vi "Stopt VI Event.vi"(2 "error in":errorcluster, 3 "VI refnum":refnum<vi>[](array[refnum])) -> (0 "error out":errorcluster)   [LabVIEW 2012]
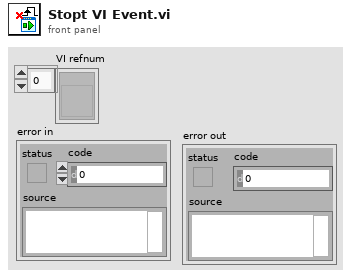
[diagram p1: front panel]
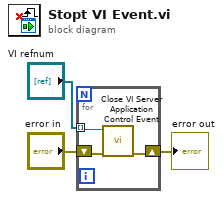
[diagram p0: block diagram]
diagram:
  n1 = for {
    tunnel: "VI refnum" -> [w6] mode=indexing
    shift-right: [w4] -> w1
    shift-left: "error in" -> [w5]
    n2 = call "Close VI Server Application Control Event.vi"("error in (no error)"=w5, "VI refnum"=w6) -> ("error out"=w4:errorcluster)  [unwired: 9 in]
  }
  "error out" <- w1
